vi "ResetConfiguration.vi"(2 "error in (no error)":errorcluster, 3 "EpiWrapper in":refnum<class "EpiWrapper.lvclass">) -> (0 "error out":errorcluster, 1 "EpiWrapper out":refnum<class "EpiWrapper.lvclass">)   [LabVIEW 2012, in "EpiWrapper.lvclass"]
uses:
  EpiWrapper.lvclass
  EpiWrapper.lvclass/EpiWrapper.ctl
  Instruments.lvclass
  Controls/Config.ctl
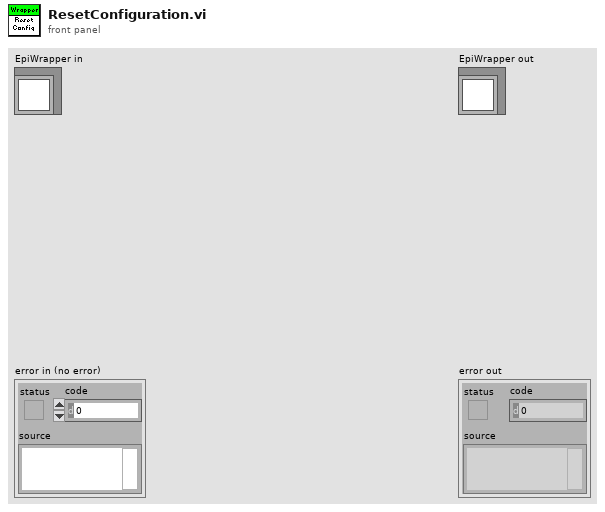
[diagram p1: front panel]
types:
  T1 = typedef "Config.ctl" = cluster{"IntTime":i32, "Samples":i32, "PowerMin":dbl, "KneeMin":dbl, "KneeMax":dbl, "BackgroundWl":dbl}
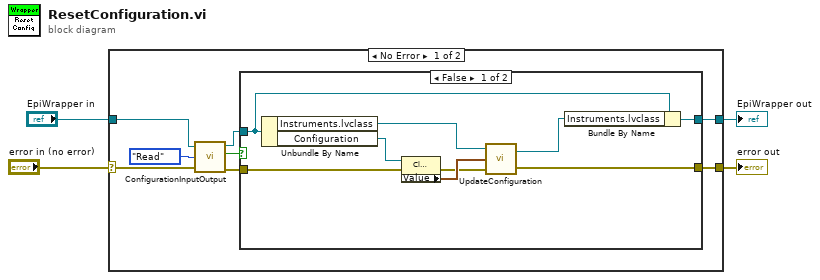
[diagram p0: block diagram]
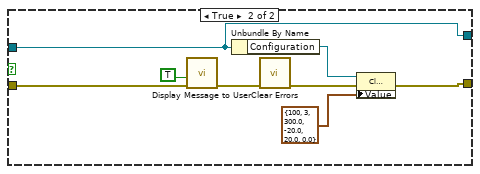
[diagram p2: hidden frame]
diagram:
  n1 = case shown="No Error" "error in (no error)" {
    selector: "error in (no error)" -> [w10 w31]
    tunnel: [w7 w31] -> w3
    tunnel: [w5 w30] -> w1
    tunnel: "EpiWrapper in" -> [w12 w30]
    frame No Error {
      n2 = call-dynamic "ConfigurationInputOutput.vi"("EpiWrapper in"=w12, "Action"=enum16{"Read", "Write"}."Read", "error in (no error)"=w10) -> ("EpiWrapper out"=w8:refnum<class "EpiWrapper.lvclass">, "error?"=w9:bool, "error out"=w6:errorcluster)  [unwired: 1 out]
      n3 = case shown="False" w9 {
        tunnel: w8 -> [w20 w27]
        tunnel: [w17 w22] -> w7
        tunnel: w6 -> [w15 w29]
        tunnel: [w18 w27] -> w5
        frame False {
          n4 = Unbundle By Name(w20) -> ("Instruments.lvclass"=w21:refnum<class "Instruments.lvclass">, "Configuration"=w16:refnum<vi>)
          n5 = property class="Clust (strict)"(reference=w16, error in=w15) -> (error out=w13:errorcluster, "Value"=w14:T1)  [unwired: 1 out]
          n6 = call-dynamic "UpdateConfiguration.vi"("error in (no error)"=w13, "Value"=w14, "Instruments in"=w21) -> ("error out"=w17:errorcluster, "Instruments out"=w19:refnum<class "Instruments.lvclass">)
          n7 = Bundle By Name(cluster=w20, "Instruments.lvclass"=w19) -> (w18:refnum<class "EpiWrapper.lvclass">)
        }
        frame True {
          n8 = call "Display Message to User"("error in (no error)"=w29, "Enable"=TRUE) -> ("error out"=w26:errorcluster)  [unwired: 8 in, 1 out]
          n9 = Unbundle By Name(w27) -> ("Configuration"=w25:refnum<vi>)
          n10 = call <vilib>:"Clear Errors.vi"("error in (no error)"=w26) -> ("error out"=w23:errorcluster)  [unwired: 6 in]
          n11 = property class="Clust (strict)"(reference=w25, error in=w23, "Value"=T1 {"IntTime"=100, "Samples"=3, "PowerMin"=300.0, "KneeMin"=-20.0, "KneeMax"=20.0, "BackgroundWl"=0.0}) -> (error out=w22:errorcluster)  [unwired: 1 out]
        }
      }
    }
    frame Error {
    }
  }
  "error out" <- w3
  "EpiWrapper out" <- w1
